vi "Build Numeric Constants.vi"   [LabVIEW 2021]
uses:
  <vilib>/numeric/LVNumericRepresentation.ctl
types:
  T1 = typedef "LVNumericRepresentation.ctl" = enum32{"Extended Precision", "Double Precision", "Single Precision", "Long", "Word", "Byte", "Unsigned Long", "Unsigned Word", "Unsigned Byte", "Complex Extended", "Complex Double", "Complex Single", "Quad", "Unsigned Quad", "Fixed-Point"}
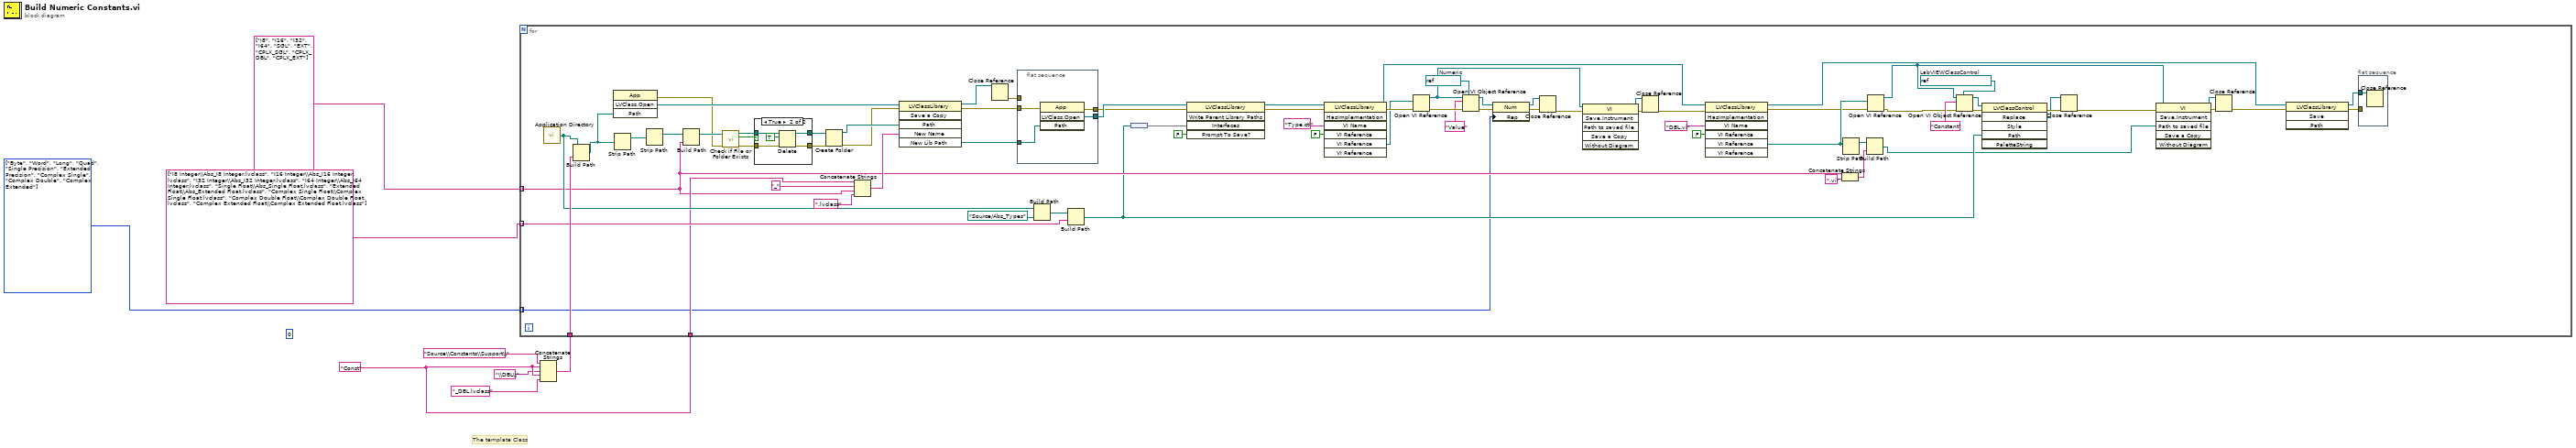
[diagram p0: block diagram]
diagram:
  (unwired) 0 ("length")
  w1 = T1[] [enum."Byte", enum."Word", enum."Long", enum."Quad", enum."Single Precision", enum."Extended Precision", enum."Complex Single", enum."Complex Double", enum."Complex Extended"] items=["Extended Precision", "Double Precision", "Single Precision", "Long", "Word", "Byte", "Unsigned Long", "Unsigned Word", "Unsigned Byte", "Complex Extended", "Complex Double", "Complex Single", "Quad", "Unsigned Quad", "Fixed-Point"] ("Representation")
  w8 = "Const" ("Comparison Name")
  # "The template Class"
  n1 = Concatenate Strings("Source\\Constants\\Support\\", w8, "\\DBL\\", w8, "_DBL.lvclass") -> (w7:string)
  n2 = for {
    tunnel: string[] ["I8", "I16", "I32", "I64", "SGL", "EXT", "CPLX_SGL", "CPLX_DBL", "CPLX_EXT"] -> [w36] mode=indexing
    tunnel: w7 -> [w64]
    tunnel: string[] ["I8 Integer\\Abs_I8 Integer.lvclass", "I16 Integer\\Abs_I16 Integer.lvclass", "I32 Integer\\Abs_I32 Integer.lvclass", "I64 Integer\\Abs_I64 Integer.lvclass", "Single Float\\Abs_Single Float.lvclass", "Extended Float\\Abs_Extended Float.lvclass", "Complex Single Float\\Complex Single Float.lvclass", "Complex Double Float\\Complex Double Float.lvclass", "Complex Extended Float\\Complex Extended Float.lvclass"] -> [w58] mode=indexing
    tunnel: w1 -> [w19] mode=indexing
    tunnel: w8 -> [w47]
    w27 = refnum<vi> refnum  # Numeric
    w41 = refnum<vi> refnum  # LabVIEWClassControl
    n3 = call <vilib>:"Application Directory.vi"() -> ("Application Directory"=w52:path)
    n4 = Build Path(base path=w52, name or relative path=w64) -> (appended path=w65:path)
    n5 = invoke class="App" method="LVClass.Open"("Path"=w65) -> (error out=w70:errorcluster, "LVClass.Open"=w83:refnum<vi>)  [unwired: 3 in, 2 out]
    n6 = Strip Path(path=w65) -> (stripped path=w81:path)  [unwired: 1 out]
    n7 = Strip Path(path=w81) -> (stripped path=w80:path)  [unwired: 1 out]
    n8 = Build Path(base path=w80, name or relative path=w36) -> (appended path=w76:path)
    n9 = call <vilib>:"Check if File or Folder Exists.vi"("error in (no error)"=w70, "path"=w76) -> ("error out"=w69:errorcluster, "file or folder exists?"=w78:bool, "dup path"=w79:path)  [unwired: 7 in]
    n10 = case shown="True" w78 {
      tunnel: w79 -> [w90 w95]
      tunnel: [w90 w93] -> w77
      tunnel: w69 -> [w89 w92]
      tunnel: [w89 w91] -> w68
      frame False {
      }
      frame True {
        n11 = Delete(path (use dialog)=w95, entire hierarchy (F)=TRUE, error in=w92) -> (deleted path=w93:path, error out=w91:errorcluster)  [unwired: 2 in, 1 out]
      }
    }
    n12 = Create Folder(path (use dialog)=w77, error in=w68) -> (created path=w75:path, error out=w67:errorcluster)  [unwired: 1 in, 1 out]
    n13 = Concatenate Strings(w47, "_", w36, ".lvclass") -> (w63:string)
    n14 = invoke class="LVClassLibrary" method="Save a Copy"(reference=w83, error in=w67, "Path"=w75, "New Name"=w63) -> (reference out=w82:refnum<vi>, error out=w71:errorcluster, "New Lib Path"=w72:path)  [unwired: 2 in, 3 out]
    n15 = Close Reference(reference=w82) -> (error out=w66:errorcluster)  [unwired: 1 in]
    n16 = flat-sequence {
      tunnel: w72 -> [w87]
      tunnel: w71 -> [w88]
      tunnel: w66 -> [_]
      tunnel: [w85] -> w56
      tunnel: [w86] -> w51
      frame #0 {
        n17 = invoke class="App" method="LVClass.Open"(error in=w88, "Path"=w87) -> (error out=w86:errorcluster, "LVClass.Open"=w85:refnum<vi>)  [unwired: 2 in, 2 out]
      }
    }
    n18 = Build Path(base path=w52, name or relative path=path "Source/Abs_Types") -> (appended path=w59:path)
    n19 = Build Path(base path=w59, name or relative path=w58) -> (appended path=w34:path)
    n20 = node(w34) -> (w50:set{path})
    n21 = invoke class="LVClassLibrary" method="Write Parent Library Paths"(reference=w56, error in=w51, "Interfaces"=w50, "Prompt To Save?"=FALSE) -> (reference out=w29:refnum<vi>, error out=w30:errorcluster)  [unwired: 1 in, 3 out]
    n22 = invoke class="LVClassLibrary" method="HasImplementation"(reference=w29, error in=w30, "VI Name"="Type.ctl", "VI Reference"=FALSE ("Consider Parents?")) -> (reference out=w12:refnum<vi>, error out=w21:errorcluster, "VI Reference"=w14:path)  [unwired: 3 in, 4 out]
    n23 = Open VI Reference(vi path=w14, error in (no error)=w21) -> (vi reference=w15:refnum<vi>, error out=w28:errorcluster)  [unwired: 4 in]
    n24 = Open VI Object Reference(7:w27, 8:w28, 10:"Value" ("name/order"), 11:w15) -> (0:w26:errorcluster, 3:w25:refnum<vi>)
    n25 = property class="Num"(reference=w25, error in=w26, "Rep"=w19) -> (reference out=w24:refnum<vi>, error out=w23:errorcluster)
    n26 = Close Reference(reference=w24, error in (no error)=w23) -> (error out=w16:errorcluster)
    n27 = invoke class="VI" method="Save.Instrument"(reference=w15, error in=w16) -> (reference out=w18:refnum<vi>, error out=w17:errorcluster)  [unwired: 4 in, 4 out]
    n28 = Close Reference(reference=w18, error in (no error)=w17) -> (error out=w13:errorcluster)
    n29 = invoke class="LVClassLibrary" method="HasImplementation"(reference=w12, error in=w13, "VI Name"="DBL.vi", "VI Reference"=FALSE ("Consider Parents?")) -> (reference out=w10:refnum<vi>, error out=w11:errorcluster, "VI Reference"=w39:path)  [unwired: 3 in, 4 out]
    n30 = Concatenate Strings(w36, ".vi" ("string")) -> (w37:string)
    n31 = Strip Path(path=w39) -> (stripped path=w38:path)  [unwired: 1 out]
    n32 = Build Path(base path=w38, name or relative path=w37) -> (appended path=w9:path)
    n33 = Open VI Reference(vi path=w39, error in (no error)=w11) -> (vi reference=w33:refnum<vi>, error out=w20:errorcluster)  [unwired: 4 in]
    n34 = Open VI Object Reference(7:w41, 8:w20, 10:"Constant" ("name/order"), 11:w33) -> (0:w45:errorcluster, 3:w46:refnum<vi>)
    n35 = invoke class="LVClassControl" method="Replace"(reference=w46, error in=w45, "Path"=w34) -> (error out=w43:errorcluster, "Replace"=w42:refnum<vi>)  [unwired: 3 in, 4 out]
    n36 = Close Reference(reference=w42, error in (no error)=w43) -> (error out=w40:errorcluster)
    n37 = invoke class="VI" method="Save.Instrument"(reference=w33, error in=w40, "Path to saved file"=w9) -> (reference out=w48:refnum<vi>, error out=w49:errorcluster)  [unwired: 3 in, 4 out]
    n38 = Close Reference(reference=w48, error in (no error)=w49) -> (error out=w57:errorcluster)
    n39 = invoke class="LVClassLibrary" method="Save"(reference=w10, error in=w57) -> (reference out=w53:refnum<vi>, error out=w54:errorcluster)  [unwired: 2 in, 2 out]
    n40 = flat-sequence {
      tunnel: w53 -> [w84]
      tunnel: w54 -> [_]
      frame #0 {
        n41 = Close Reference(reference=w84) -> ()  [unwired: 1 in, 1 out]
      }
    }
  }
